vi "Data Conversion - Signed 32 Bit 1D Array to 2D Array.vi"(9 "Channels":i32, 10 "1D Data (Multiplexed)":i32[](array[numeric])) -> (2 "2D Data (De-Multiplexed)":i32[][](array[numeric]))   [LabVIEW 2017, in "Communications Library.lvlib"]
doc: "Reformats a 1D array, into a 2D array, according to the number of channels present."
uses:
  Communications Library.lvlib
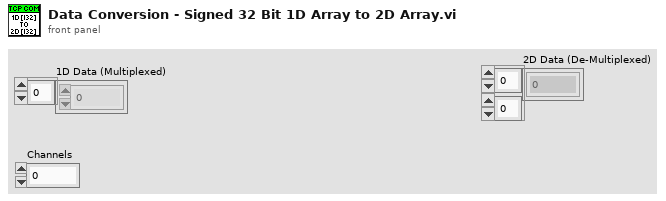
[diagram p1: front panel]
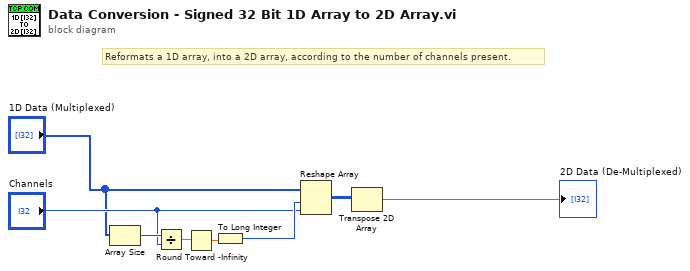
[diagram p0: block diagram]
diagram:
  # "Reformats a 1D array, into a 2D array, according to the number of channels present."
  n1 = Array Size(array="1D Data (Multiplexed)") -> (size(s)=w4:i32)
  n2 = Divide(x=w4, y="Channels") -> (x/y=w5:dbl)
  n3 = Round Toward -Infinity(1:w5) -> (0:w6:dbl)
  n4 = To Long Integer(number=w6) -> (32bit integer=w7:i32)
  n5 = Reshape Array("1D Data (Multiplexed)", w7, "Channels") -> (w8:i32[][])
  n6 = Transpose 2D Array(2D array=w8) -> (transposed array=→"2D Data (De-Multiplexed)":i32[][])
